vi "Destructor.vi"(11 "data value reference":T1) -> ()   [LabVIEW 2016, in "Impulse Data.lvclass"]
uses:
  Impulse Data.lvclass
  Instance handle.ctl
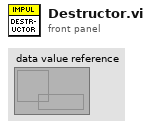
[diagram p1: front panel]
types:
  T1 = typedef "Impulse Data.lvclass/Instance handle.ctl" = refnum<data-value>
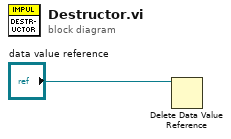
[diagram p0: block diagram]
diagram:
  n1 = Delete Data Value Reference(data value reference="data value reference") -> ()  [unwired: 1 in, 2 out]
